vi "main OP150-2.vi"() -> ()   [LabVIEW 2020]
uses:
  SubVI/OP150ZP_state.ctl
  <userlib>/Alex.vi/FGV.ctl
  <vilib>/QMT/GDataBase for MySQL(tm)/MySQL/public/controls/DateType.ctl
  Lib/02 SLIM ZEN WS 500/SubVi/VG_progressBar.vi
  SubVI/CheminDeBase.vi
  <vilib>/Utility/error.llb/Error Cluster From Error Code.vi
  OP150/VG/PN.vi
  OP150 - Copie/SubVI/VG_HYDRAU.vi
  OP150/VG/VG_BT3562.vi
  <vilib>/QMT/GDataBase for MySQL(tm)/MySQL/MySQLConnector.lvclass
panel:
  out "ATEQ":refnum<visa-resource-name>
  out "Revision":i32
  out "error out":errorcluster
  in  "arrêt":bool
  in  "last?":bool
  out "VISA OUT 2":T1
  out "Cluster 2":T2
  out "BDD":T3
  out "progression":u8(slide) scale=0.0..100.0
  out "PN":string
  out "errout 2":errorcluster={"status"=TRUE, "code"=0, "source"="PCAN_CHANNEL ILLEGAL"} caption="errout"
  out "errout":errorcluster caption="sortie d'erreur"
  out "STOP":bool
  out "TOP":string
  out "DRAW":picture
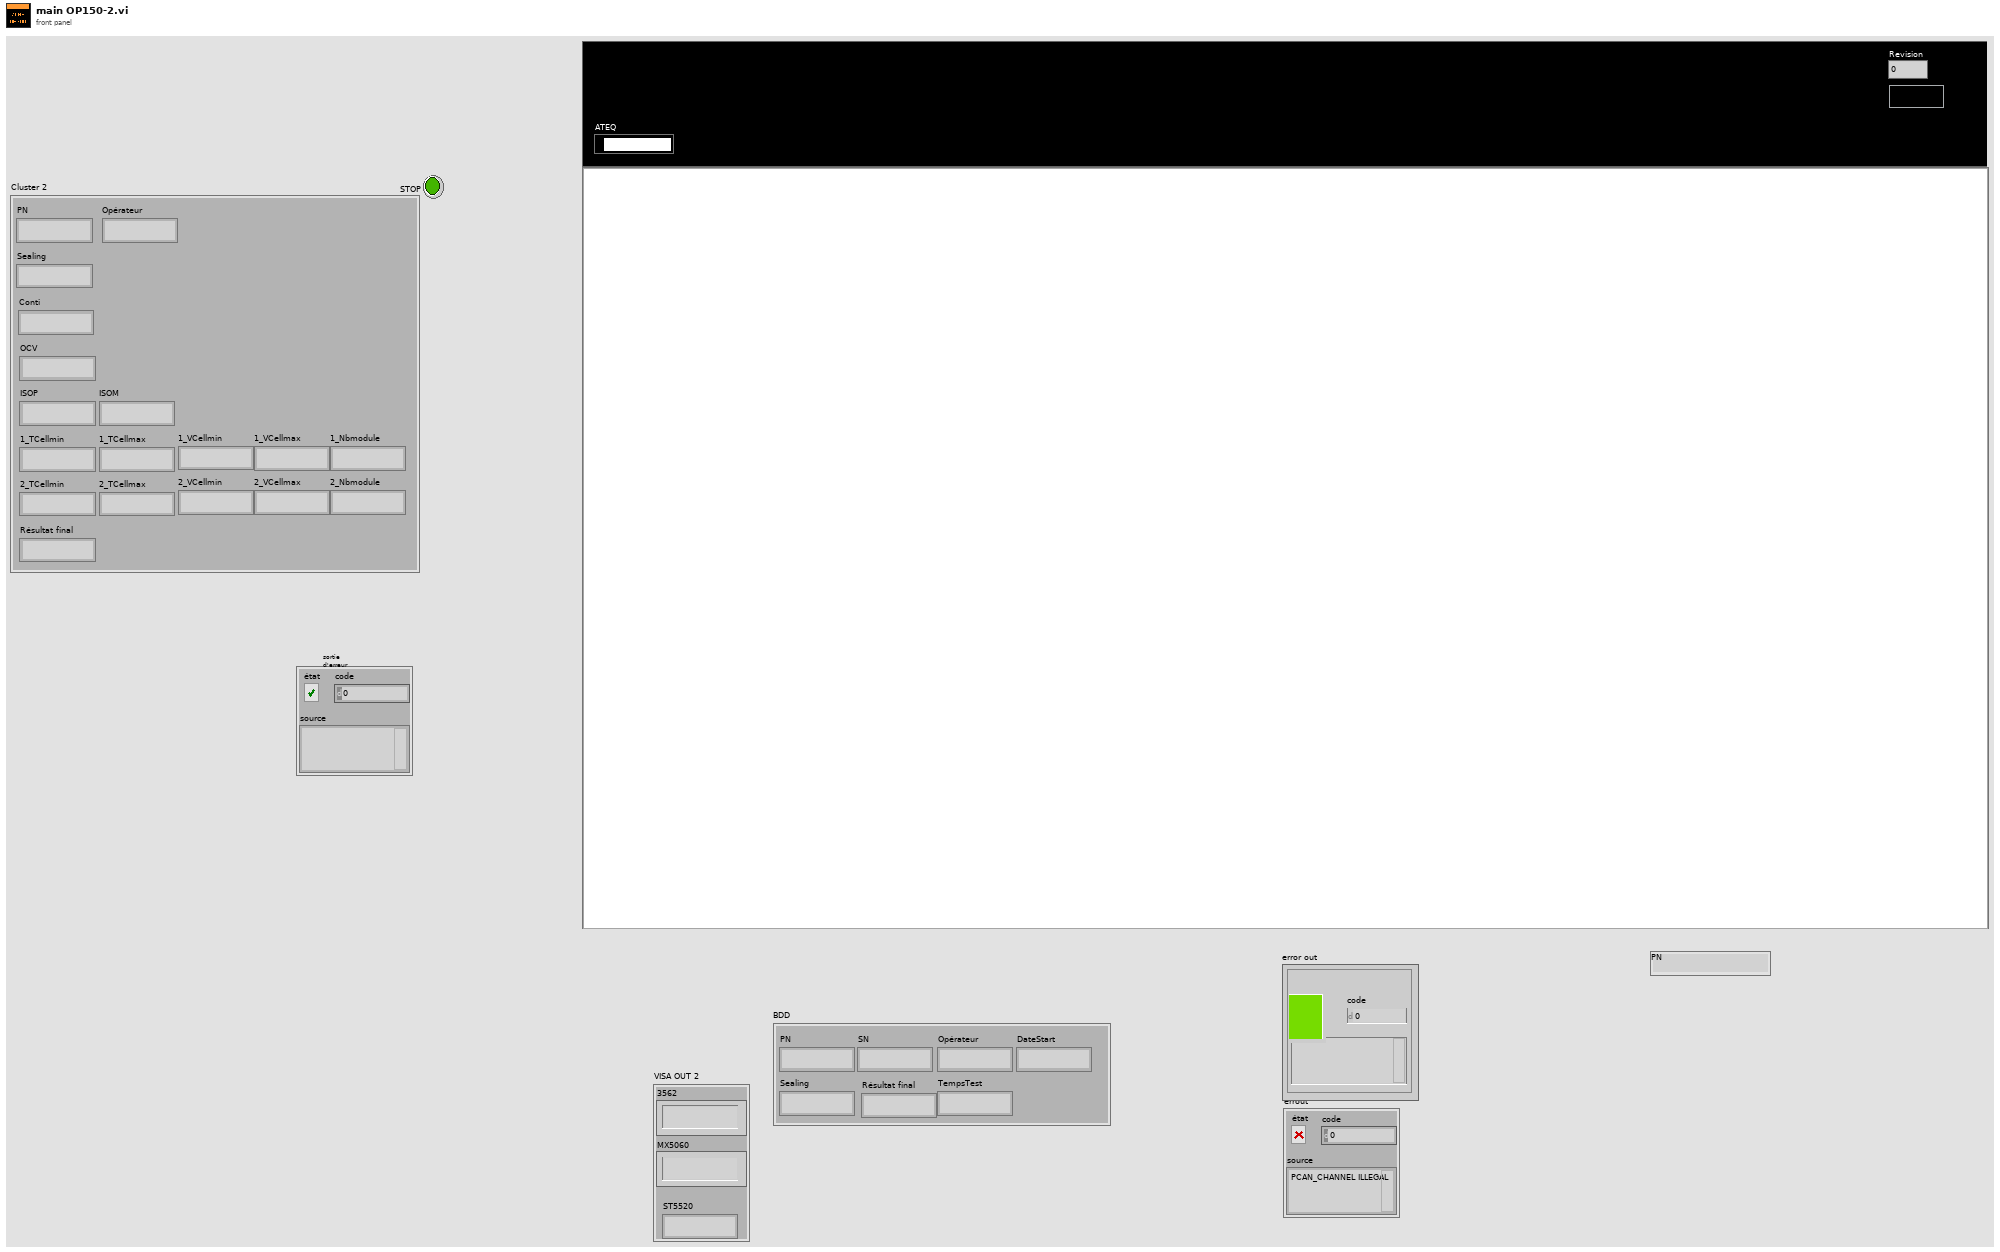
[diagram p1: front panel]
types:
  T1 = cluster{"3562":string, "MX5060":string, "ST5520":string}
  T2 = cluster{"PN":string, "Opérateur":string, "Sealing":string, "Conti":string, "OCV":string, "ISOP":string, "ISOM":string, "1_TCellmin":string, "1_TCellmax":string, "1_VCellmin":string, "1_VCellmax":string, "1_Nbmodule":string, "2_TCellmin":string, "2_TCellmax":string, "2_VCellmin":string, "2_VCellmax":string, "2_Nbmodule":string, "Résultat final":string}
  T3 = cluster{"PN":string, "Opérateur":string, "Sealing":string, "Résultat final":string, "SN":string, "DateStart":string, "TempsTest":string}
  T4 = cluster{"PN":string, "Sealing":string, "Opérateur":string, "Conti":string, "OCV":string, "ISOP":string, "ISOP 2":string}
  T5 = typedef "OP150ZP_state.ctl" = enum16{"Null", "Demarrage", "Init", "Scan", "Crash", "Next", "Conti", "Sealing", "Comext", ""}
  T6 = typedef "FGV.ctl" = enum16{"GET", "SET", "RAZ"}
  T7 = typedef "MySQLVIEW.lvlib/MySQLConnector.lvclass/DateType.ctl" = enum16{"DATETIME", "DATE", "TIMESTAMP", "TIME", "YEAR (2 digits)", "YEAR (4 digits)"}
  T8 = enum32{"BT3561A", "BT3562A", "BT3563A", "BT3562", "BT3563", "BT3564", "3561"}
  T9 = typedef "imagedata.ctl" = cluster{"image type":i32, "image depth":i32, "image":u8[], "mask":u8[], "colors":u32[], "Rectangle":cluster{"left":i16, "top":i16, "right":i16, "bottom":i16}}
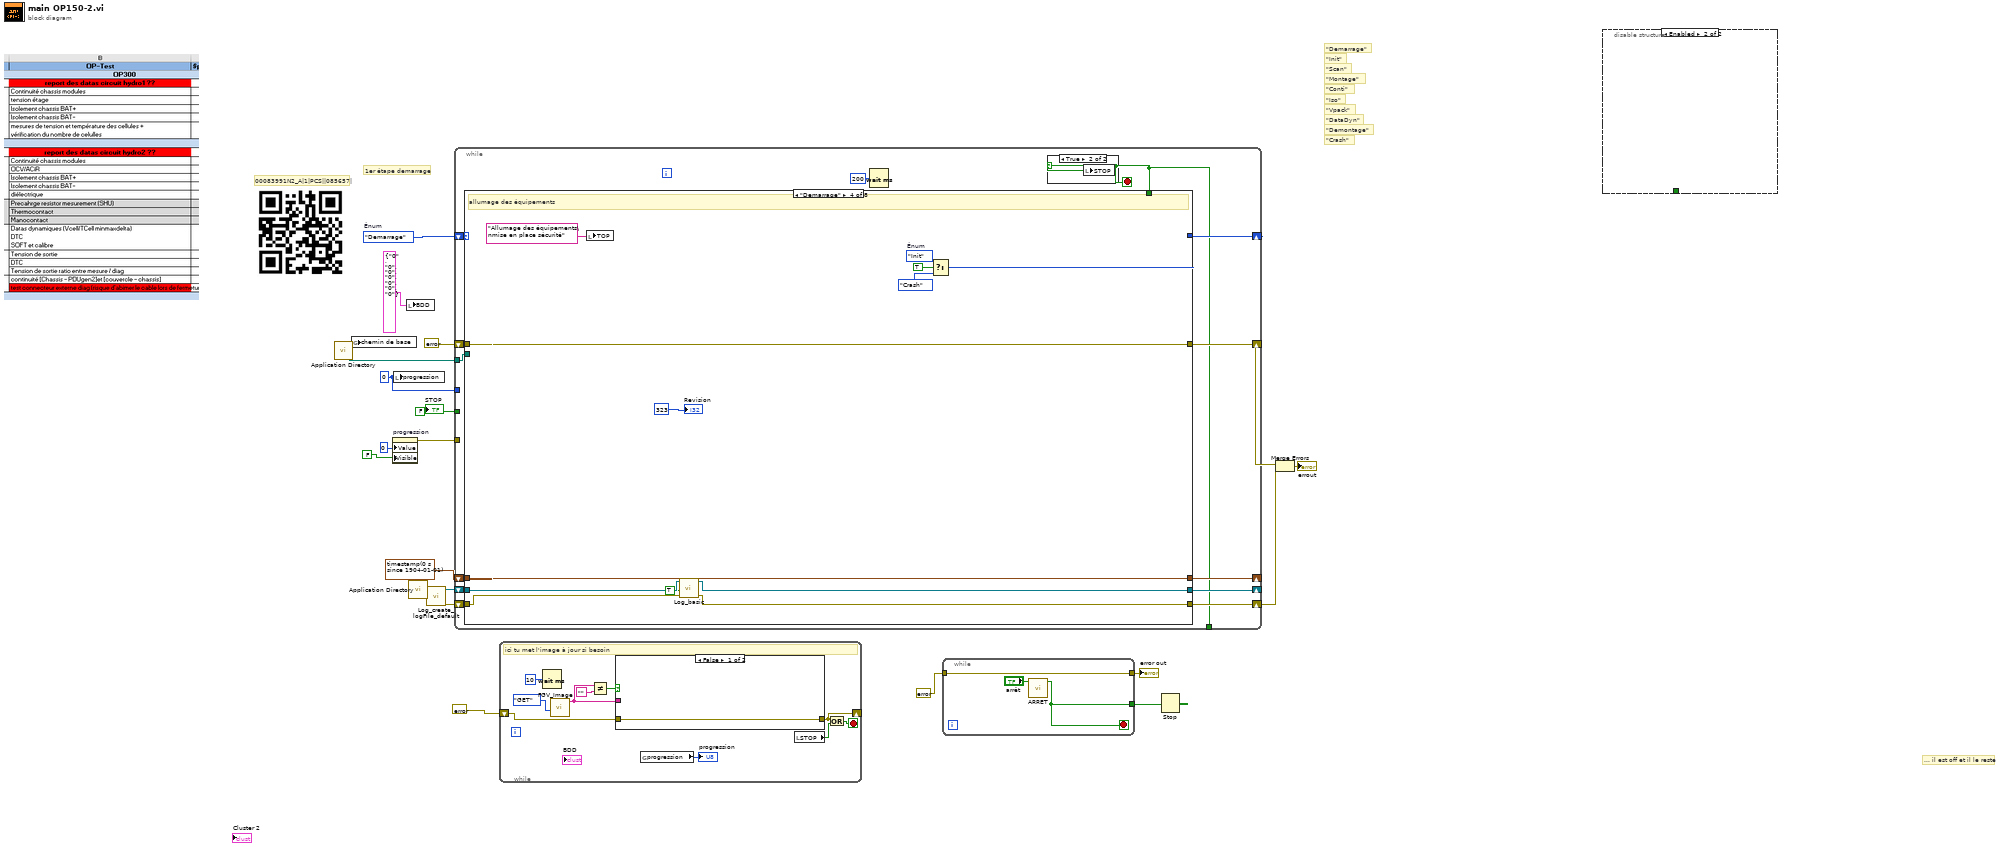
[diagram p0: block diagram]
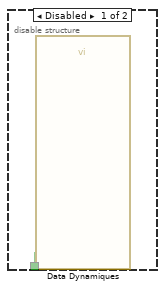
[diagram p2: hidden frame]
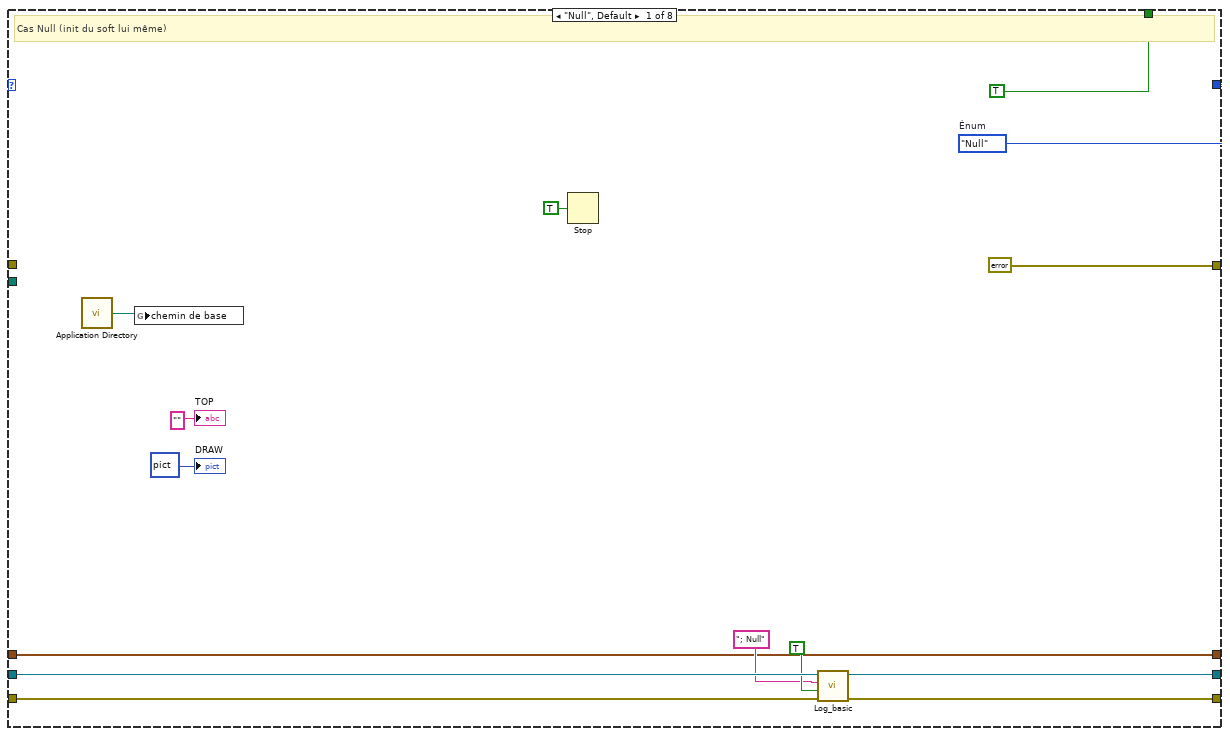
[diagram p4: hidden frame]
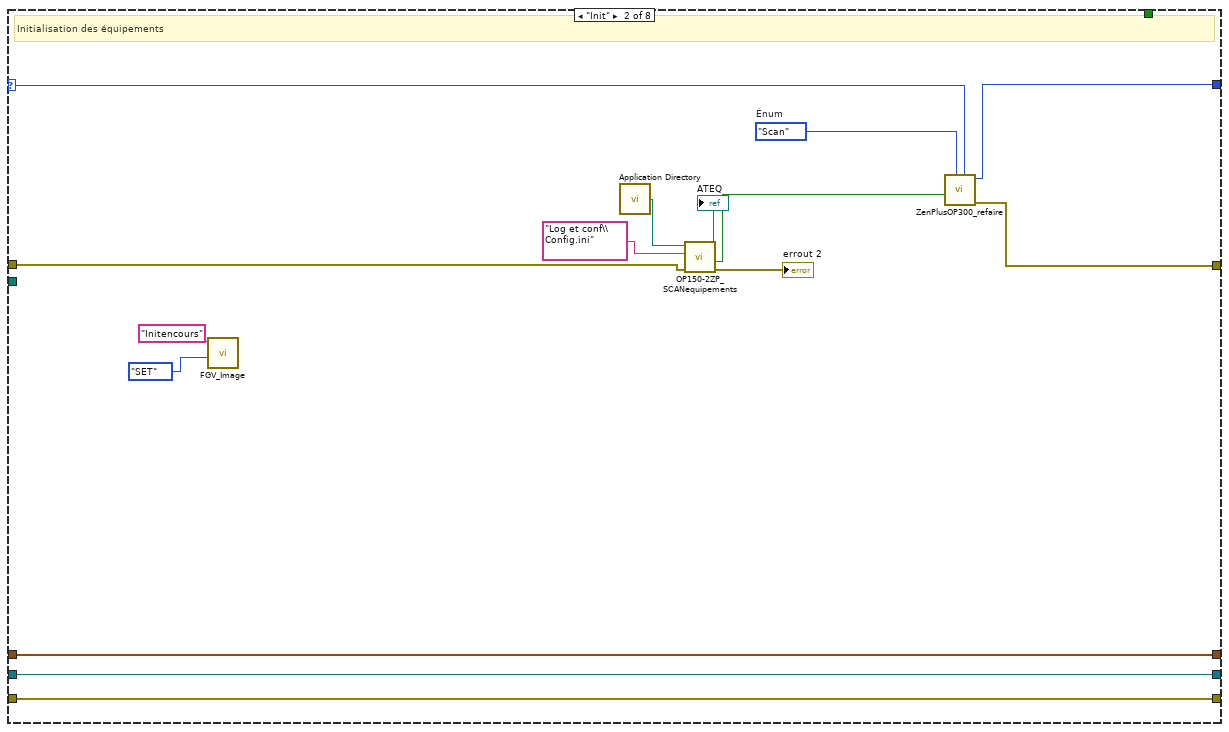
[diagram p5: hidden frame]
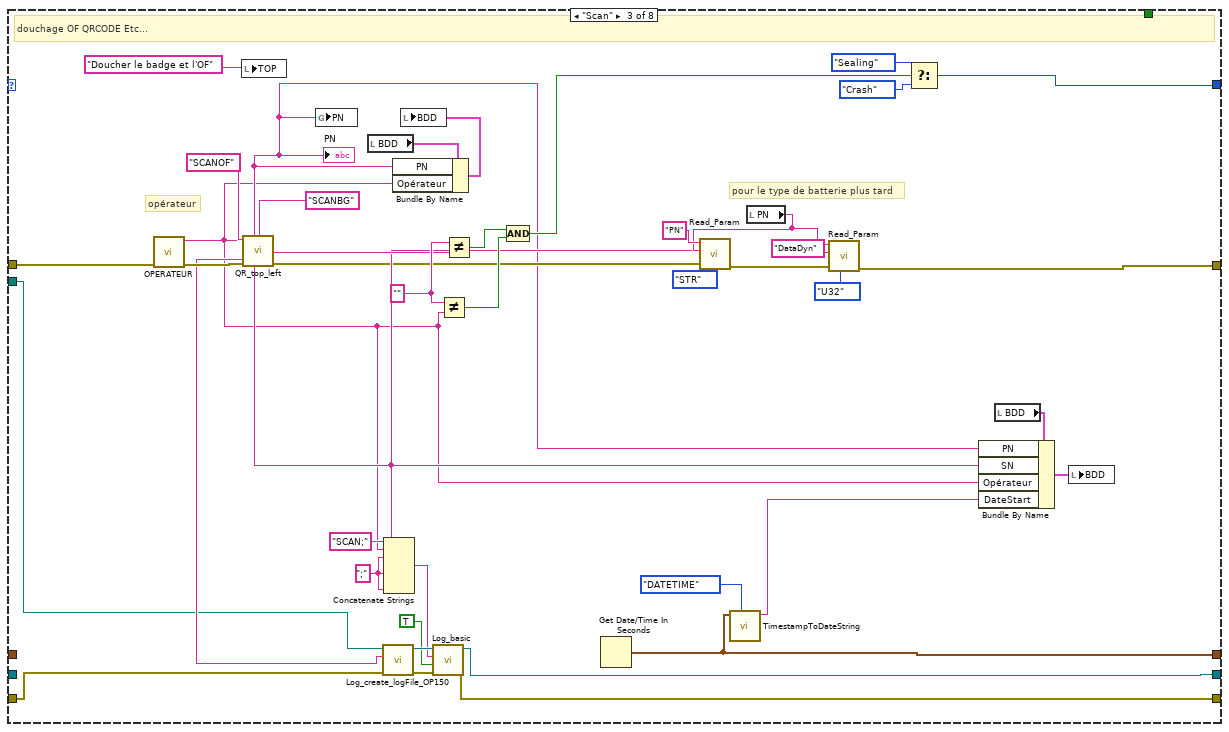
[diagram p6: hidden frame]
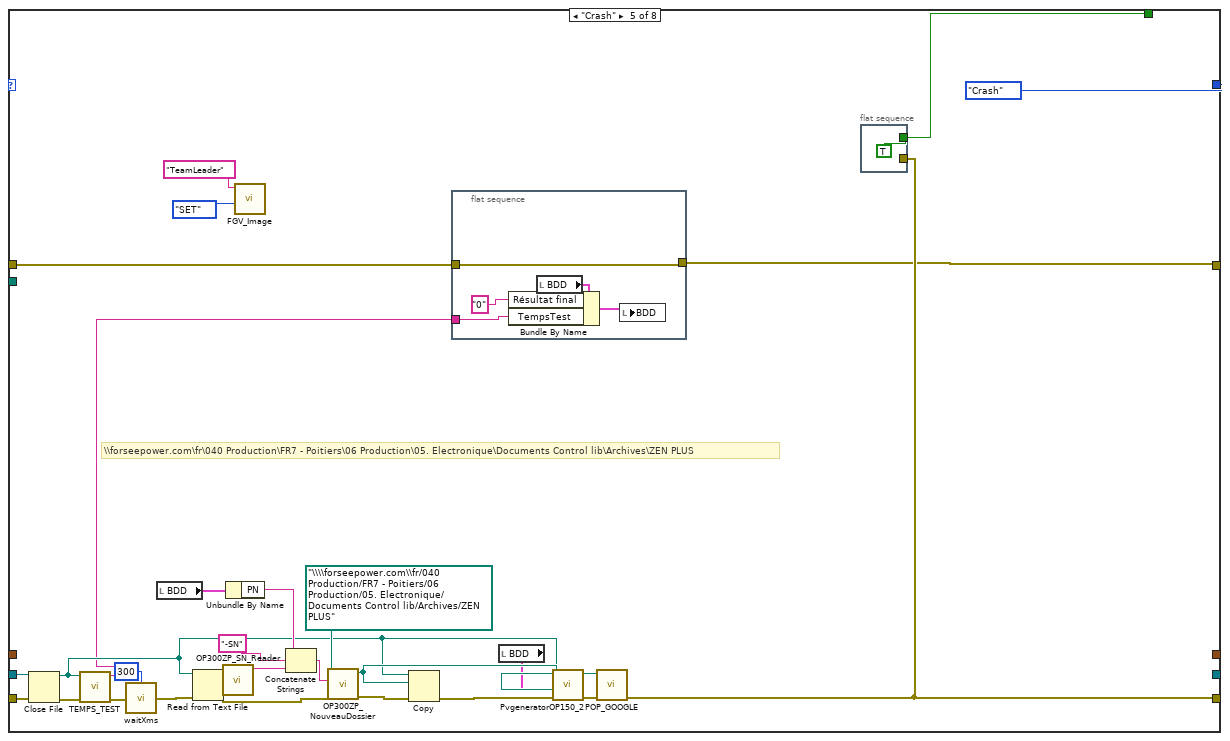
[diagram p7: hidden frame]
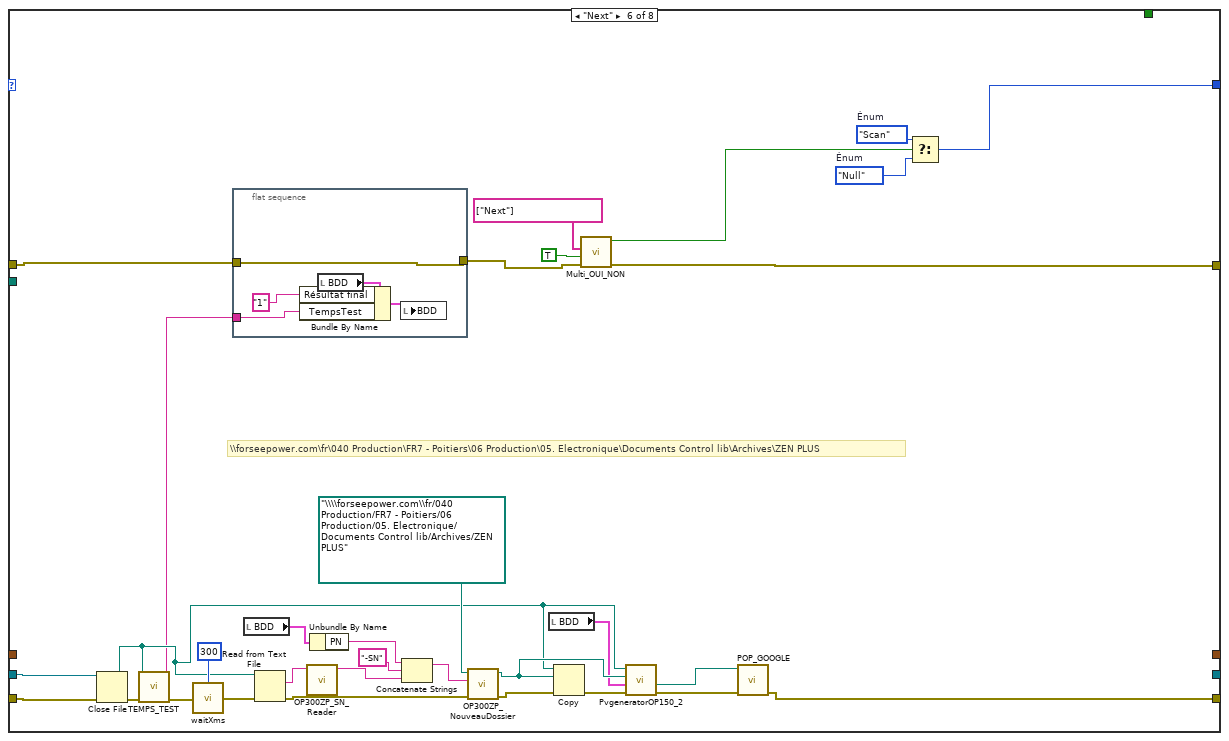
[diagram p8: hidden frame]
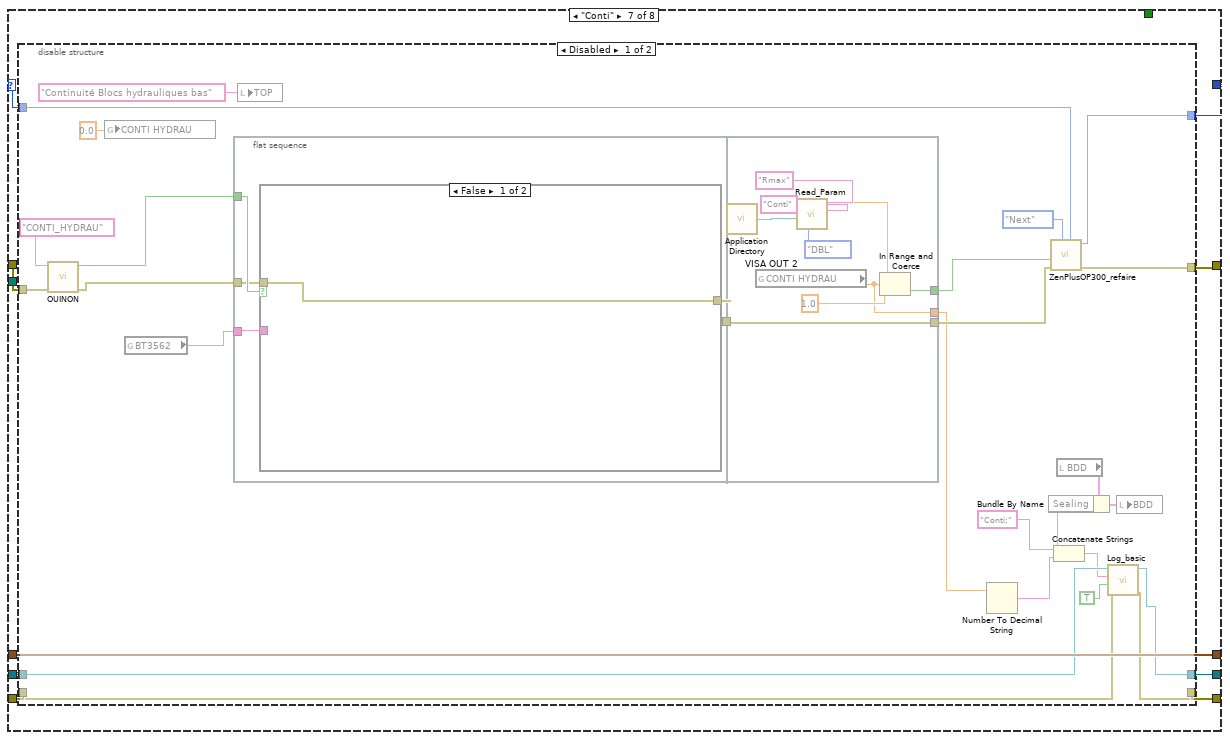
[diagram p9: hidden frame]
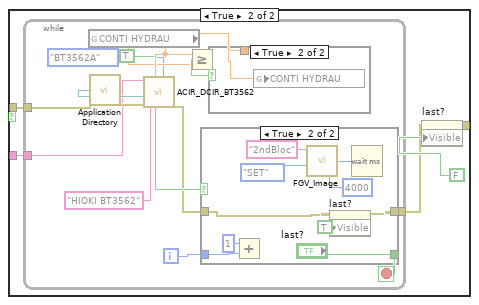
[diagram p10: hidden frame]
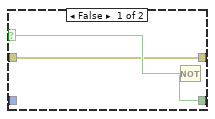
[diagram p11: hidden frame]
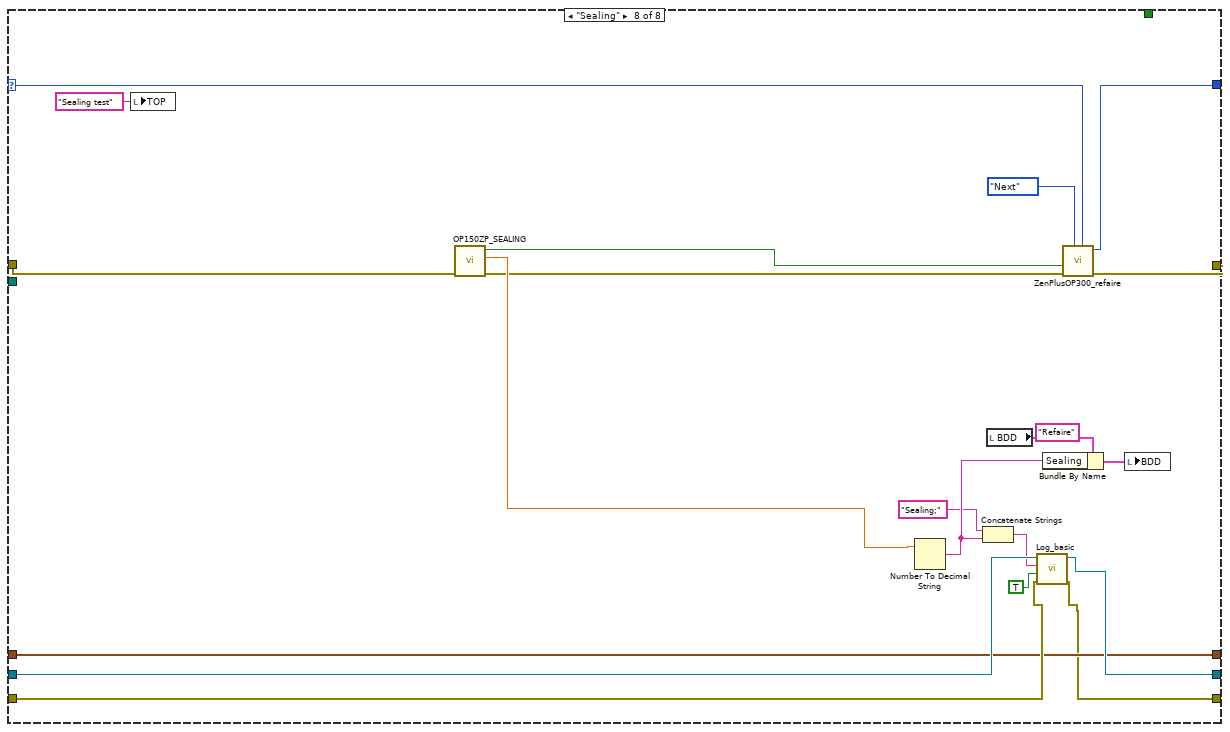
[diagram p14: hidden frame]
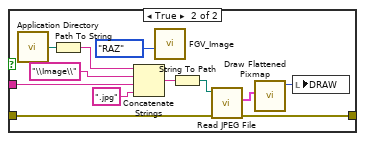
[diagram p15: hidden frame]
diagram:
  w10 = u8 0 ("progression")
  w11 = OP150ZP_state."Demarrage"  # Énum
  w17 = FALSE ("STOP")
  # "00083991N2_A|1|PCS||085657|"
  # "1er étape demarrage"
  # "\"Crash\""
  # "\"Demontage\""
  # "\"DataDyn\""
  # "\"Iso\""
  # "\"Montage\""
  # "\"Scan\""
  # "\"Init\""
  # "\"Demarrage\""
  # "\"Conti\""
  # "\"Vpack\""
  # "... il est off et il le reste"
  n1 = call <vilib>:"Application Directory.vi"() -> ("Application Directory"=w16:path)
  n2 = global write "CheminDeBase.vi" "chemin de base"(w16) -> ()
  n3 = property on="progression" class="Slide (strict)"("Value"=u8 0 ("progression"), "Visible"=FALSE) -> (error out=w8:errorcluster)  [unwired: 2 in, 1 out]
  n4 = local write "progression"(w10) -> ()
  n5 = local write "BDD"(T4 {"PN"="0", "Sealing"="0", "Opérateur"="0", "Conti"="0", "OCV"="0", "ISOP"="0", "ISOP 2"="0"} ("Cluster")) -> ()
  n6 = call <vilib>:"Application Directory.vi"() -> ("Application Directory"=w14:path)
  n7 = call "Log_create_logFile_default.vi"("appdir"=w14) -> ("errout"=w15:errorcluster, "Fichier à flux d'octets en sortie"=w18:refnum<file>)  [unwired: 9 in]
  n8 = while {
    shift-right: [w32] -> w3
    shift-left: errorcluster {"status"=FALSE, "code"=0, "source"=""} ("error out") -> [w23]
    shift-right: [w22] -> _
    shift-left: w11 -> [w27]
    shift-right: [w28] -> w19
    shift-left: w15 -> [w31]
    shift-right: [w29] -> _
    shift-left: w18 -> [w30]
    tunnel: w16 -> [w26]
    tunnel: w17 -> [_]
    shift-right: [w24] -> _
    shift-left: timestamp(0 s since 1904-01-01) ("seconds since 1Jan1904") -> [w25]
    tunnel: w10 -> [_]
    tunnel: w8 -> [_]
    tunnel: [w21] -> _
    stop <- w21 stop-if-true
    n9 = case shown="\"Demarrage\"" w27 {
      selector: w27 -> [_ w58 _ _ _ _ w198 w283]
      tunnel: w23 -> [_ w60 w105 w113 w124 w161 w199 w282]
      tunnel: [errorcluster {"status"=FALSE, "code"=0, "source"=""} ("errin") w59 w88 w113 w123 w165 w191 w287] -> w32
      tunnel: w31 -> [w44 w63 w102 w110 w145 w184 w196 w290]
      tunnel: w30 -> [w45 w62 _ w108 w146 w185 w194 w289]
      tunnel: [w42 w62 w103 w107 _ _ w193 w288] -> w29
      tunnel: [w43 w63 w104 w109 w137 w178 w195 w285] -> w28
      tunnel: [TRUE _ _ _ w147 _ _ _] -> w21
      tunnel: w26 -> [_ _ w64 _ _ _ _ _]
      tunnel: w25 -> [w38 w61 _ w118 _ _ w192 w286]
      tunnel: [w38 w61 w68 w118 _ _ w192 w286] -> w24
      tunnel: [w36 w50 w73 w114 OP150ZP_state."Crash" w162 w197 w284] -> w22
      frame "Null", Default {
        w36 = OP150ZP_state."Null"  # Énum
        # "Cas Null (init du soft lui même)"
        n10 = call <vilib>:"Application Directory.vi"() -> ("Application Directory"=w48:path)
        n11 = global write "CheminDeBase.vi" "chemin de base"(w48) -> ()
        n12 = Stop(stop? (T)=TRUE) -> ()
        n13 = call "Log_basic.vi"("errin"=w44, "date?"=TRUE, "chaîne"="; Null", "in"=w45) -> ("sortie d'erreur"=w43:errorcluster, "refnum en sortie"=w42:refnum<file>)  [unwired: 6 in]
        "DRAW" <- picture data[5B] ("DRAW")
        "TOP" <- "" ("TOP")
      }
      frame "Init" {
        w54 = OP150ZP_state."Scan"  # Énum
        # "Initialisation des équipements"
        n14 = call <userlib>:"FGV_Image.vi"("Énum"=FGV."SET", "IN"="Initencours") -> ()  [unwired: 8 in, 2 out]
        n15 = call <vilib>:"Application Directory.vi"() -> ("Application Directory"=w51:path)
        n16 = call "OP150-2ZP_SCANequipements.vi"("Errin"=w60, "Chaîne"="Log et conf\\Config.ini", "pathin"=w51) -> ("ERROUT"=→"errout 2":errorcluster, "KO?"=w55:bool, "ATEQ"=→"ATEQ":refnum<visa-resource-name>)  [unwired: 6 in]
        n17 = call "ZenPlusOP300_refaire.vi"("refaire"=w58, "casOK"=w54, "test ok ?"=w55) -> ("errout"=w59:errorcluster, "Next"=w50:T5)  [unwired: 7 in]
      }
      frame "Scan" {
        w74 = ";" ("chaîne")
        w96 = "" ("x")
        # "pour le type de batterie plus tard"
        # "opérateur"
        # "douchage OF QRCODE Etc..."
        n18 = call "OPERATEUR.vi"("errin"=w105, "IN"="SCANBG") -> ("error out"=w93:errorcluster, "Dataout"=w69:string)  [unwired: 8 in]
        n19 = local write "TOP"("Doucher le badge et l'OF" ("TOP")) -> ()
        n20 = call <userlib>:"QR_top_left.vi"("errin"=w93, "image"="SCANOF") -> ("error out"=w75:errorcluster, "Réponse"=w91:string, "SN"=w70:string, "PN"=w71:string)  [unwired: 5 in, 1 out]
        "PN" <- w71
        n21 = global write "PN.vi" "PN"(w71) -> ()
        n22 = local read "BDD"() -> (w77:T3)
        n23 = call "Log_create_logFile_OP150.vi"("errin"=w102, "toute l'expression"=w70, "Application Directory"=w64) -> ("sortie d'erreur"=w100:errorcluster, "Fichier à flux d'octets en sortie"=w101:refnum<file>)  [unwired: 7 in]
        n24 = Bundle By Name(cluster=w77, "PN"=w71, "Opérateur"=w69) -> (w76:T3)
        n25 = local write "BDD"(w76) -> ()
        n26 = Not Equal?(x=w96, y=w69) -> (x != y?=w94:bool)
        n27 = Not Equal?(x=w96, y=w91) -> (x != y?=w95:bool)
        n28 = Compound Arithmetic op=AND ("Opérateur arithmétique")(w95, w94) -> (w81:bool)
        n29 = Get Date/Time In Seconds() -> (seconds since 1Jan1904=w68:timestamp)
        n30 = call <vilib>:"TimestampToDateString.vi"("dateType"=DateType."DATETIME", "timestamp in"=w68) -> ("dateString"=w67:string)  [unwired: 8 in, 1 out]
        n31 = local read "PN"() -> (w84:string)
        n32 = call <userlib>:"Read_Param.vi"("Énum"=enum16{"STR", "DBL", "U32"}."STR", "errin"=w75, "section"=w84, "key"="PN") -> ("error out"=w87:errorcluster, "str"=w83:string)  [unwired: 3 in, 3 out]
        n33 = Concatenate Strings("SCAN;" ("chaîne"), w69, w74, w70, w74, w83, w74) -> (w98:string)
        n34 = call "Log_basic.vi"("errin"=w100, "date?"=TRUE, "chaîne"=w98, "in"=w101) -> ("sortie d'erreur"=w104:errorcluster, "refnum en sortie"=w103:refnum<file>)  [unwired: 6 in]
        n35 = call <userlib>:"Read_Param.vi"("Énum"=enum16{"STR", "DBL", "U32"}."U32", "errin"=w87, "section"="DataDyn", "key"=w84) -> ("error out"=w88:errorcluster)  [unwired: 3 in, 4 out]
        n36 = Select ("Sélectionner")(t=OP150ZP_state."Sealing" ("Énum"), s=w81, f=OP150ZP_state."Crash" ("cas faux")) -> (s? t:f=w73:T5)
        n37 = local read "BDD"() -> (w72:T3)
        n38 = Bundle By Name(cluster=w72, "PN"=w71, "SN"=w70, "Opérateur"=w69, "DateStart"=w67) -> (w66:T3)
        n39 = local write "BDD"(w66) -> ()
      }
      frame "Demarrage" {
        w116 = OP150ZP_state."Init"  # Énum
        # "allumage des équipements"
        n40 = local write "TOP"("Allumage des équipements\nmise en place sécurité" ("TOP")) -> ()
        n41 = call "Log_basic.vi"("errin"=w110, "date?"=TRUE, "in"=w108) -> ("sortie d'erreur"=w109:errorcluster, "refnum en sortie"=w107:refnum<file>)  [unwired: 7 in]
        n42 = Select ("Sélectionner")(t=w116, s=TRUE, f=OP150ZP_state."Crash" ("cas faux")) -> (s? t:f=w114:T5)
        "Revision" <- 323
      }
      frame "Crash" {
        # "\\\\forseepower.com\\fr\\040 Production\\FR7 - Poitiers\\06 Production\\05. Electronique\\Documents Control lib\\Archives\\ZEN PLUS"
        n43 = Close File(refnum=w146, error in=w145) -> (path=w121:path, error out=w139:errorcluster)
        n44 = call <userlib>:"TEMPS_TEST.vi"("errin"=w139, "pathin"=w121) -> ("error out"=w122:errorcluster, "Delay calculé"=w120:string)  [unwired: 8 in]
        n45 = call <userlib>:"waitXms.vi"("attente (ms)"=u32 300, "errin"=w122) -> ("errout"=w136:errorcluster)  [unwired: 13 in]
        n46 = local read "BDD"() -> (w130:T3)
        n47 = Read from Text File(file (use dialog)=w121, error in=w136) -> (text=w135:string, error out=w133:errorcluster)  [unwired: 2 in, 2 out]
        n48 = call "OP300ZP_SN_Reader.vi"("Fichier txt"=w135) -> ("SN"=w128:string)  [unwired: 10 in]
        n49 = Unbundle By Name(w130) -> ("PN"=w127:string)
        n50 = call <userlib>:"FGV_Image.vi"("Énum"=FGV."SET", "IN"="TeamLeader") -> ()  [unwired: 8 in, 2 out]
        n51 = Concatenate Strings(w127, "-SN" ("chaîne"), w128) -> (w129:string)
        n52 = call "OP300ZP_NouveauDossier.vi"("entrée d'erreur (pas d'erreur)"=w133, "Nom du repertoire (PN SN)"=w129, "Network before adding a new folder"=path "\\\\forseepower.com\\fr/040 Production/FR7 - Poitiers/06 Production/05. Electronique/Documents Control lib/Archives/ZEN PLUS" ("chemin de la cible (utiliser une boîte de dialogue)")) -> ("sortie d'erreur"=w134:errorcluster, "Network after adding a new folder"=w131:path)  [unwired: 7 in]
        n53 = Copy ("Copier")(8:w134, 10:w131, 11:w121) -> (0:w138:errorcluster)  [unwired: 2 in, 2 out]
        n54 = flat-sequence {
          tunnel: [w150] -> w123
          tunnel: w124 -> [w150]
          tunnel: w120 -> [w148]
          frame #0 {
            n55 = local read "BDD"() -> (w152:T3)
            n56 = Bundle By Name(cluster=w152, "Résultat final"="0", "TempsTest"=w148) -> (w149:T3)
            n57 = local write "BDD"(w149) -> ()
          }
        }
        n58 = local read "BDD"() -> (w119:T3)
        n59 = call "PvgeneratorOP150_2.vi"("errin"=w138, "BDD"=w119, "network"=w131, "path in"=w121) -> ("sortie d'erreur"=w142:errorcluster, "network out"=w141:path)  [unwired: 4 in, 2 out]
        n60 = call "POP_GOOGLE.vi"("error in"=w142, "chemin"=w141) -> ("error out"=w137:errorcluster)  [unwired: 8 in, 1 out]
        n61 = flat-sequence {
          tunnel: [TRUE] -> w147
          tunnel: w137 -> [_]
          frame #0 {
          }
        }
      }
      frame "Next" {
        w182 = OP150ZP_state."Null"  # Énum
        w183 = OP150ZP_state."Scan"  # Énum
        # "\\\\forseepower.com\\fr\\040 Production\\FR7 - Poitiers\\06 Production\\05. Electronique\\Documents Control lib\\Archives\\ZEN PLUS"
        n62 = Close File(refnum=w185, error in=w184) -> (path=w158:path, error out=w159:errorcluster)
        n63 = call <userlib>:"TEMPS_TEST.vi"("errin"=w159, "pathin"=w158) -> ("error out"=w156:errorcluster, "Delay calculé"=w155:string)  [unwired: 8 in]
        n64 = call <userlib>:"waitXms.vi"("attente (ms)"=u32 300, "errin"=w156) -> ("errout"=w157:errorcluster)  [unwired: 13 in]
        n65 = flat-sequence {
          tunnel: [w188] -> w160
          tunnel: w161 -> [w188]
          tunnel: w155 -> [w186]
          frame #0 {
            n66 = local read "BDD"() -> (w190:T3)
            n67 = Bundle By Name(cluster=w190, "Résultat final"="1", "TempsTest"=w186) -> (w187:T3)
            n68 = local write "BDD"(w187) -> ()
          }
        }
        n69 = local read "BDD"() -> (w171:T3)
        n70 = Read from Text File(file (use dialog)=w158, error in=w157) -> (text=w176:string, error out=w175:errorcluster)  [unwired: 2 in, 2 out]
        n71 = call "OP300ZP_SN_Reader.vi"("Fichier txt"=w176) -> ("SN"=w168:string)  [unwired: 10 in]
        n72 = Unbundle By Name(w171) -> ("PN"=w170:string)
        n73 = Concatenate Strings(w170, "-SN" ("chaîne"), w168) -> (w167:string)
        n74 = call "OP300ZP_NouveauDossier.vi"("entrée d'erreur (pas d'erreur)"=w175, "Nom du repertoire (PN SN)"=w167, "Network before adding a new folder"=path "\\\\forseepower.com\\fr/040 Production/FR7 - Poitiers/06 Production/05. Electronique/Documents Control lib/Archives/ZEN PLUS" ("chemin de la cible (utiliser une boîte de dialogue)")) -> ("sortie d'erreur"=w174:errorcluster, "Network after adding a new folder"=w172:path)  [unwired: 7 in]
        n75 = local read "BDD"() -> (w154:T3)
        n76 = Copy ("Copier")(8:w174, 10:w172, 11:w158) -> (0:w177:errorcluster)  [unwired: 2 in, 2 out]
        n77 = call "Multi_OUI_NON.vi"("errin"=w160, "errinb"=TRUE, "Tableau"=string[] ["Next"]) -> ("errout"=w165:errorcluster, "isok?"=w164:bool)  [unwired: 7 in]
        n78 = call "PvgeneratorOP150_2.vi"("errin"=w177, "BDD"=w154, "network"=w172, "path in"=w158) -> ("sortie d'erreur"=w180:errorcluster, "network out"=w179:path)  [unwired: 4 in, 2 out]
        n79 = call "POP_GOOGLE.vi"("error in"=w180, "chemin"=w179) -> ("error out"=w178:errorcluster)  [unwired: 8 in, 1 out]
        n80 = Select(t=w183, s=w164, f=w182) -> (s? t:f=w162:T5)
      }
      frame "Conti" {
        n81 = disable-structure shown="Disabled" {
          disable-tunnel: w199 -> [w223 _]
          disable-tunnel: w198 -> [w222 _]
          disable-tunnel: [w221 _] -> w197
          disable-tunnel: w196 -> [w220 _]
          disable-tunnel: [w219 _] -> w195
          disable-tunnel: w194 -> [w218 _]
          disable-tunnel: [w217 _] -> w193
          disable-tunnel: [w216 _] -> w191
          frame Disabled {
            n82 = call "OUINON.vi"("errin"=w223, "image"="CONTI_HYDRAU" ("IN")) -> ("error out"=w207:errorcluster, "OUI/NON"=w212:bool)  [unwired: 8 in]
            n83 = global write "VG_HYDRAU.vi" "CONTI HYDRAU"(0.0 ("R")) -> ()
            n84 = global read "VG_BT3562.vi" "BT3562"() -> (w206:string)
            n85 = flat-sequence {
              tunnel: w212 -> [w228]
              tunnel: w206 -> [w227]
              tunnel: w207 -> [w226]
              tunnel: [w225] -> w224
              tunnel: [w264] -> w208
              tunnel: [w263] -> w209
              tunnel: [w262] -> w210
              tunnel: w224 -> [w262]
              frame #0 {
                n86 = case shown="False" w228 {
                  tunnel: w227 -> [_ w234]
                  tunnel: w226 -> [w229 w233]
                  tunnel: [w229 w231] -> w225
                  frame False {
                  }
                  frame True {
                    n87 = while {
                      tunnel: w234 -> [w238]
                      tunnel: w233 -> [w248]
                      tunnel: [w245] -> w230
                      i -> [w244]
                      stop <- w241 stop-if-true
                      n88 = global read "VG_HYDRAU.vi" "CONTI HYDRAU"() -> (w239:dbl)
                      n89 = call <vilib>:"Application Directory.vi"() -> ("Application Directory"=w247:path)
                      n90 = call <userlib>:"ACIR_DCIR_BT3562.vi"("Model"=T8."BT3562A", "juste R?"=TRUE, "errin"=w248, "chemin de base"=w247, "section"="HIOKI BT3562", "VISAin"=w238) -> ("errout"=w240:errorcluster, "OK?"=w246:bool, "R"=w242:dbl)  [unwired: 3 out]
                      n91 = Greater Or Equal?(x=w242, y=w239) -> (x >= y?=w243:bool)
                      n92 = case shown="True" w246 {
                        selector: w246 -> [w251 _]
                        tunnel: w240 -> [w249 w253]
                        tunnel: [w249 w255] -> w245
                        tunnel: [w250 "last?"] -> w241
                        tunnel: w244 -> [_ w258]
                        frame False {
                          n93 = Not(x=w251) -> (.not. x?=w250:bool)
                        }
                        frame True {
                          n94 = Add(x=1, y=w258) -> ()  [unwired: 1 out]
                          n95 = call <userlib>:"FGV_Image.vi"("Énum"=FGV."SET", "IN"="2ndBloc") -> ()  [unwired: 8 in, 2 out]
                          n96 = property on="last?" class="Bool"(error in=w253, "Visible"=TRUE) -> (error out=w255:errorcluster)  [unwired: 1 in, 1 out]
                          n97 = Wait (ms)(milliseconds to wait=u32 4000 ("attente (ms)")) -> ()  [unwired: 1 out]
                        }
                      }
                      n98 = case shown="True" w243 {
                        tunnel: w242 -> [_ w261]
                        frame False {
                        }
                        frame True {
                          n99 = global write "VG_HYDRAU.vi" "CONTI HYDRAU"(w261) -> ()
                        }
                      }
                    }
                    n100 = property on="last?" class="Bool"(error in=w230, "Visible"=FALSE) -> (error out=w231:errorcluster)  [unwired: 1 in, 1 out]
                  }
                }
              }
              frame #1 {
                n101 = call <vilib>:"Application Directory.vi"() -> ("Application Directory"=w268:path)
                n102 = global read "VG_HYDRAU.vi" "CONTI HYDRAU"() -> (w263:dbl)
                n103 = call <userlib>:"Read_Param.vi"("Énum"=enum16{"STR", "DBL", "U32"}."DBL", 9:w268, "section"="Conti", "key"="Rmax") -> ("dbl"=w266:dbl)  [unwired: 3 in, 4 out]
                n104 = In Range and Coerce(upper limit=w266, x=w263, lower limit=1.0 ("limite inférieure")) -> (In Range?=w264:bool)  [unwired: 1 out]
              }
            }
            n105 = local write "TOP"("Continuité Blocs hydrauliques bas" ("TOP")) -> ()
            n106 = Number To Decimal String(number=w209) -> (decimal integer string=w203:string)  [unwired: 1 in]
            n107 = call "ZenPlusOP300_refaire.vi"("refaire"=w222, "casOK"=OP150ZP_state."Next" ("refaire"), "errin"=w210, "test ok ?"=w208) -> ("errout"=w216:errorcluster, "Next"=w221:T5)  [unwired: 6 in]
            n108 = Concatenate Strings("Conti;" ("chaîne"), w203) -> (w201:string)
            n109 = local read "BDD"() -> (w204:T3)
            n110 = Bundle By Name(cluster=w204, "Sealing"=w203) -> (w205:T3)
            n111 = call "Log_basic.vi"("errin"=w220, "date?"=TRUE, "chaîne"=w201, "in"=w218) -> ("sortie d'erreur"=w219:errorcluster, "refnum en sortie"=w217:refnum<file>)  [unwired: 6 in]
            n112 = local write "BDD"(w205) -> ()
          }
          frame Enabled {
          }
        }
      }
      frame "Sealing" {
        (unwired) "Refaire" ("image")
        n113 = local write "TOP"("Sealing test" ("TOP")) -> ()
        n114 = call "OP150ZP_SEALING.vi"("ERRIN"=w282) -> ("ERROUT"=w271:errorcluster, "SEALING_VALUE"=w276:dbl, "IsOK?"=w272:bool)  [unwired: 8 in]
        n115 = Number To Decimal String(number=w276) -> (decimal integer string=w279:string)  [unwired: 1 in]
        n116 = Concatenate Strings("Sealing;" ("chaîne"), w279) -> (w274:string)
        n117 = local read "BDD"() -> (w281:T3)
        n118 = call "Log_basic.vi"("errin"=w290, "date?"=TRUE, "chaîne"=w274, "in"=w289) -> ("sortie d'erreur"=w285:errorcluster, "refnum en sortie"=w288:refnum<file>)  [unwired: 6 in]
        n119 = Bundle By Name(cluster=w281, "Sealing"=w279) -> (w280:T3)
        n120 = call "ZenPlusOP300_refaire.vi"("refaire"=w283, "casOK"=OP150ZP_state."Next" ("refaire"), "errin"=w271, "test ok ?"=w272) -> ("errout"=w287:errorcluster, "Next"=w284:T5)  [unwired: 6 in]
        n121 = local write "BDD"(w280) -> ()
      }
    }
    n122 = Wait (ms)(milliseconds to wait=u32 200 ("attente (ms)")) -> ()  [unwired: 1 out]
    n123 = case shown="True" w21 {
      selector: w21 -> [_ w34]
      frame False {
      }
      frame True {
        n124 = local write "STOP"(w34) -> ()
      }
    }
  }
  n125 = while {
    shift-right: [w299] -> _
    shift-left: errorcluster {"status"=FALSE, "code"=0, "source"=""} ("error out") -> [w296]
    stop <- w297 stop-if-true
    # "ici tu met l'image à jour si besoin"
    n126 = Wait (ms)(milliseconds to wait=u32 10 ("attente (ms)")) -> ()  [unwired: 1 out]
    n127 = call <userlib>:"FGV_Image.vi"("Énum"=FGV."GET") -> ("OUT"=w292:string)  [unwired: 9 in, 1 out]
    n128 = Not Equal?(x=w292, y="") -> (x != y?=w293:bool)
    n129 = case shown="False" w293 {
      tunnel: [w301 w306] -> w299
      tunnel: w296 -> [w301 w305]
      tunnel: w292 -> [_ w304]
      frame False {
      }
      frame True {
        n130 = call <vilib>:"Application Directory.vi"() -> ("Application Directory"=w309:path)
        n131 = Path To String(path=w309) -> (string=w310:string)
        n132 = Concatenate Strings(w310, "\\Image\\" ("chaîne"), w304, ".jpg" ("chaîne")) -> (w308:string)
        n133 = call <userlib>:"FGV_Image.vi"("Énum"=FGV."RAZ") -> ()  [unwired: 9 in, 2 out]
        n134 = String To Path(string=w308) -> (path=w307:path)
        n135 = call <vilib>:"Read JPEG File.vi"("error in (no error)"=w305, "path to JPEG file"=w307) -> ("error out"=w306:errorcluster, "image data"=w313:T9)  [unwired: 7 in, 1 out]
        n136 = call <vilib>:"Draw Flattened Pixmap.vi"("image data"=w313) -> ("new picture"=w302:picture)  [unwired: 8 in]
        n137 = local write "DRAW"(w302) -> ()
      }
    }
    n138 = global read "VG_progressBar.vi" "progression"() -> (→"progression":u8)
    n139 = local read "STOP"() -> (w298:bool)
    n140 = Or(x=w299, y=w298) -> (x .or. y?=w297:bool)
  }
  n141 = while {
    tunnel: [w315] -> w4
    tunnel: errorcluster {"status"=FALSE, "code"=0, "source"=""} ("error out") -> [w315]
    tunnel: [w314] -> w2
    stop <- w314 stop-if-true
    n142 = call "ARRET.vi"("arrêt"="arrêt") -> ("T button?"=w314:bool)  [unwired: 10 in]
  }
  "error out" <- w4
  n143 = Stop(stop? (T)=w2) -> ()
  n144 = Merge Errors(w3, w19) -> (→"errout":errorcluster)
  n145 = disable-structure shown="Enabled" {
    disable-tunnel: [w317 _] -> _
    frame Disabled {
      n146 = call "Data Dynamiques"() -> ("CMU OK"=w317:bool)  [unwired: 12 in, 7 out]
    }
    frame Enabled {
    }
  }
  "STOP" <- w17
